vi "tt20panel_handle_error.vi"(8 "error in (no error)":errorcluster, 11 "tt20panel in":refnum<class "tt20panel.lvclass">) -> (0 "error out":errorcluster, 3 "tt20panel out":refnum<class "tt20panel.lvclass">)   [LabVIEW 2015, in "tt20panel.lvclass"]
uses:
  tt20panel.lvclass
  tt20panel.lvclass/tt20panel.ctl
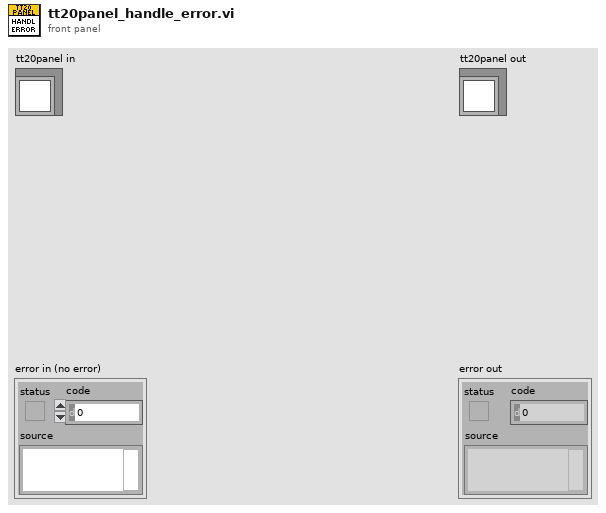
[diagram p1: front panel]
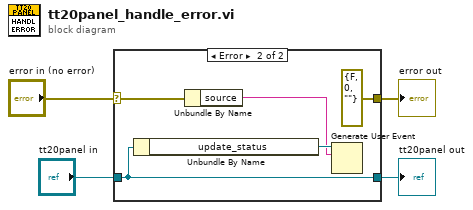
[diagram p0: block diagram]
diagram:
  n1 = case shown="Error" "error in (no error)" {
    selector: "error in (no error)" -> [w5 w11]
    tunnel: [w5 errorcluster {"status"=FALSE, "code"=0, "source"=""} ("error IO")] -> w3
    tunnel: [w6 w10] -> w1
    tunnel: "tt20panel in" -> [w6 w10]
    frame No Error {
    }
    frame Error {
      n2 = Unbundle By Name(w10) -> ("update_status"=w9:refnum<user-event>)
      n3 = Unbundle By Name(w11) -> ("source"=w8:string)
      n4 = Generate User Event(user event=w9, event data cluster=w8) -> ()  [unwired: 2 in, 2 out]
    }
  }
  "error out" <- w3
  "tt20panel out" <- w1
